vi "Configure Remote Instrument.vi"(0 "VISA resource name":refnum<visa-resource-name>="TCPIP::10.0.42.55::1394::SOCKET", 5 "Action (0: Lock)":u16(ring) items=["Lock", "Unlock", "Set New Password"], 9 "Password (Empty)":string, 11 "error in (no error)":errorcluster) -> (4 "VISA resource name out":refnum<visa-resource-name>, 15 "error out":errorcluster)   [LabVIEW 2020, in "Keithley 27XX.lvlib"]
doc: "This VI is used to configure the password options for the Model 2701 multimeter. \n\nNote:\n(1) From the front panel, the password can be cleared. When cleared the use of password is disabled and the password name resets to \"DEFAULT\". The password can be cleared using the SETUP menu as follows:\n Press SHIFT\n Press SETUP\n Use the edit keys to display CLR PASSWORD: N or Y(Clear)\n Press ENTER"
uses:
  Keithley 27XX.lvlib
panel:
  # "This VI only works with the Keithley Model 2701"
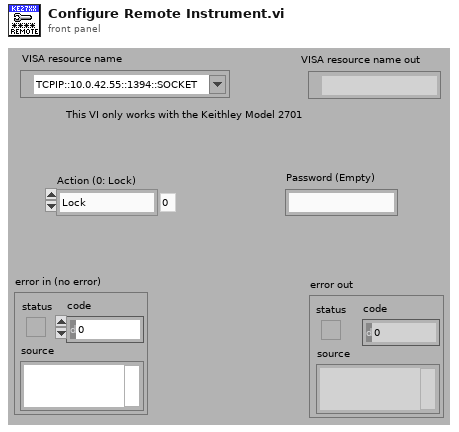
[diagram p1: front panel]
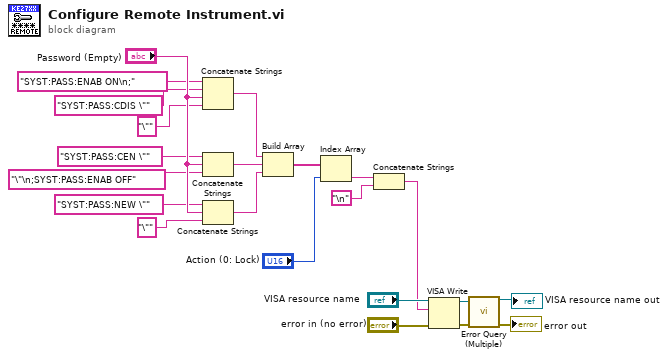
[diagram p0: block diagram]
diagram:
  n1 = Concatenate Strings("SYST:PASS:ENAB ON\n;", "SYST:PASS:CDIS \"", "Password (Empty)", "\"") -> (w13:string)
  n2 = Concatenate Strings("SYST:PASS:CEN \"", "Password (Empty)", "\"\n;SYST:PASS:ENAB OFF") -> (w12:string)
  n3 = Concatenate Strings("SYST:PASS:NEW \"", "Password (Empty)", "\"") -> (w11:string)
  n4 = Build Array(w13, w12, w11) -> (w10:string[])
  n5 = Index Array(array=w10, index="Action (0: Lock)") -> (element=w8:string)
  n6 = Concatenate Strings(w8, "\n") -> (w14:string)
  n7 = VISA Write(VISA resource name="VISA resource name", write buffer=w14, error in (no error)="error in (no error)") -> (VISA resource name out=w19:refnum<visa-resource-name>, error out=w18:errorcluster)  [unwired: 1 out]
  n8 = call "Error Query (Multiple).vi"("VISA resource name"=w19, "error in (no error)"=w18) -> ("VISA resource name out"=→"VISA resource name out":refnum<visa-resource-name>, "error out"=→"error out":errorcluster)  [unwired: 10 in, 2 out]
